vi "Wave Write.vi"(8 "error in":errorcluster, 9 "Audio Input (+/- 1)":dbl[](array[numeric]), 10 "Sound Format":T1={"sound quality"=enum."mono", "rate"=44100} {"rate" min=4000 step=1000}, 11 "File Path":path) -> (0 "error out":errorcluster)   [LabVIEW 2014]
doc: "Stores waveform data and its sound format information into a file."
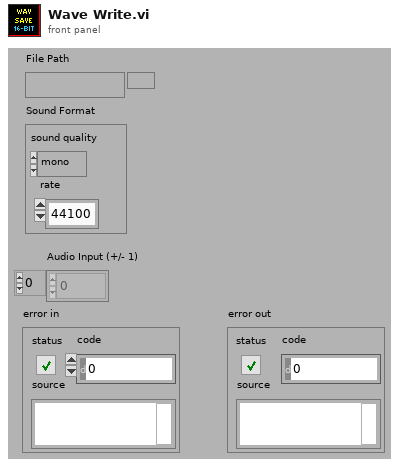
[diagram p1: front panel]
types:
  T1 = cluster{"sound quality":enum16{"mono", "stereo"}, "rate":u32}
  T2 = enum16{"big-endian, network order", "native, host order", "little-endian"}
  T3 = enum16{"open", "replace", "create", "open or create", "replace or create", "replace or create with confirmation"}
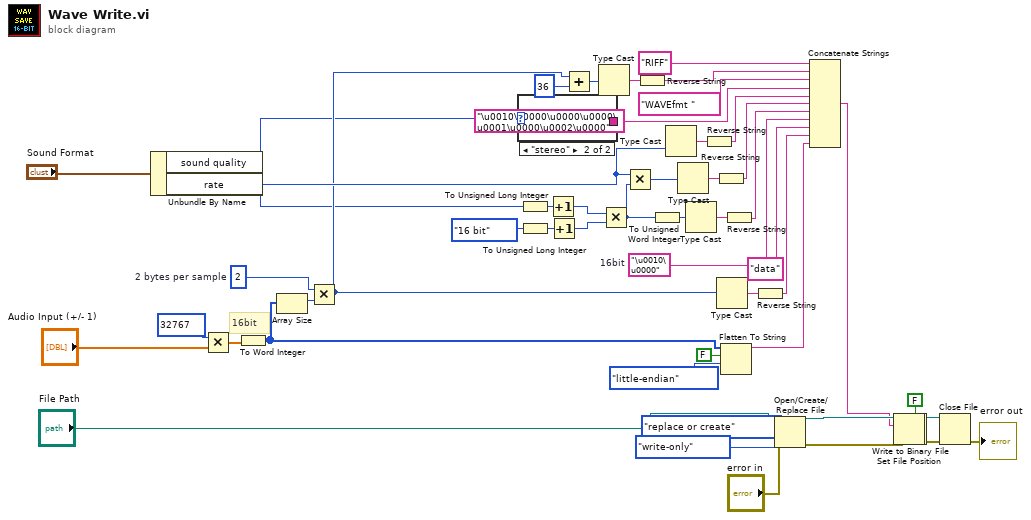
[diagram p0: block diagram]
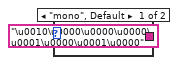
[diagram p2: hidden frame]
diagram:
  w8 = 2  # 2 bytes per sample
  w29 = "\u0010\u0000"  # 16bit
  # "16bit"
  n1 = Unbundle By Name("Sound Format") -> ("sound quality"=w7:enum16{"mono", "stereo"}, "rate"=w24:u32)
  n2 = Multiply(x=i16 32767 ("samples"), y="Audio Input (+/- 1)") -> (x*y=w6:dbl[])
  n3 = To Word Integer(number=w6) -> (16bit integer=w12:i16[])
  n4 = Array Size(array=w12) -> (size(s)=w11:i32)
  n5 = Multiply(x=w8, y=w11) -> (x*y=w10:i32)
  n6 = case shown="\"stereo\"" w7 {
    tunnel: ["\u0010\u0000\u0000\u0000\u0001\u0000\u0001\u0000" "\u0010\u0000\u0000\u0000\u0001\u0000\u0002\u0000"] -> w30
    frame "mono", Default {
    }
    frame "stereo" {
    }
  }
  n7 = To Unsigned Long Integer(number=w7) -> (unsigned 32bit integer=w40:u32)
  n8 = To Unsigned Long Integer(number=enum16{"8 bit", "16 bit"}."16 bit" ("bits per sample")) -> (unsigned 32bit integer=w39:u32)
  n9 = Increment(x=w40) -> (x+1=w38:u32)
  n10 = Increment(x=w39) -> (x+1=w37:u32)
  n11 = Add(x=w10, y=36) -> (x+y=w46:i32)
  n12 = Type Cast(x=w46) -> (*(type *) &x=w48:string)  [unwired: 1 in]
  n13 = Multiply(x=w38, y=w37) -> (x*y=w35:u32)
  n14 = Multiply(x=w24, y=w35) -> (x*y=w9:u32)
  n15 = Reverse String(1:w48) -> (0:w45:string)
  n16 = To Unsigned Word Integer(number=w35) -> (unsigned 16bit integer=w34:u16)
  n17 = Type Cast(x=w24) -> (*(type *) &x=w44:string)  [unwired: 1 in]
  n18 = Type Cast(x=w9) -> (*(type *) &x=w42:string)  [unwired: 1 in]
  n19 = Type Cast(x=w34) -> (*(type *) &x=w36:string)  [unwired: 1 in]
  n20 = Reverse String(1:w44) -> (0:w43:string)
  n21 = Reverse String(1:w42) -> (0:w41:string)
  n22 = Type Cast(x=w10) -> (*(type *) &x=w49:string)  [unwired: 1 in]
  n23 = Flatten To String(anything=w12, prepend array or string size? (T)=FALSE, byte order (0:big-endian, network order)=T2."little-endian") -> (data string=w17:string)  [unwired: 1 in, 2 out]
  n24 = Reverse String(1:w36) -> (0:w33:string)
  n25 = Reverse String(1:w49) -> (0:w31:string)
  n26 = Open/Create/Replace File(file path (use dialog)="File Path", error in="error in", operation (0:open)=T3."replace or create", access (0:read/write)=enum16{"read/write", "read-only", "write-only"}."write-only") -> (refnum out=w28:refnum<file>, error out=w26:errorcluster)  [unwired: 2 in, 1 out]
  n27 = Concatenate Strings("RIFF", w45, "WAVEfmt ", w30, w43, w41, w33, w29, "data", w31, w17) -> (w19:string)
  n28 = Set File Position(refnum=w28, error in=w26) -> (refnum out=w23:refnum<file>, error out=w22:errorcluster)  [unwired: 2 in]
  n29 = Write to Binary File(file (use dialog)=w23, data=w19, error in=w22, 5:FALSE ("prepend array or string size? (T)")) -> (refnum out=w27:refnum<file>, error out=w25:errorcluster)  [unwired: 2 in, 1 out]
  n30 = Close File(refnum=w27, error in=w25) -> (error out=→"error out":errorcluster)  [unwired: 1 out]
